vi "Compile Analog Replay Voltage Scaling.vi"(7 "DAC bipolar range":dbl, 8 "error in (no error)":errorcluster, 11 "Item Ref in":T1 format="%.0x") -> (0 "error out":errorcluster, 1 "intercept (b)":fxp<+/-,18,3>, 2 "slope (m)":fxp<+,18,6>, 3 "Item Ref out":T1 format="%.0x")   [LabVIEW 2019, in "Engine Simulation Toolkit System Explorer.lvlib"]
uses:
  Engine Simulation Toolkit System Explorer.lvlib
  <vilib>/NI VeriStand/Custom Device API/Custom Device Item Ref.ctl
  Shared/Properties.vi
  <vilib>/NI VeriStand/Custom Device API/Get Item Property (Double).vi
  <vilib>/NI VeriStand/Custom Device API/Custom Device API.lvlib
  Shared/Engine Simulation Toolkit Shared.lvlib
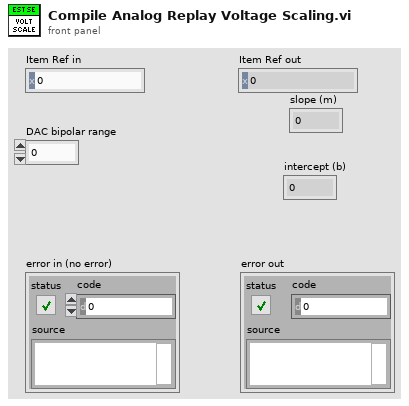
[diagram p1: front panel]
types:
  T1 = typedef "Custom Device API.lvlib/Custom Device Item Ref.ctl" = u64
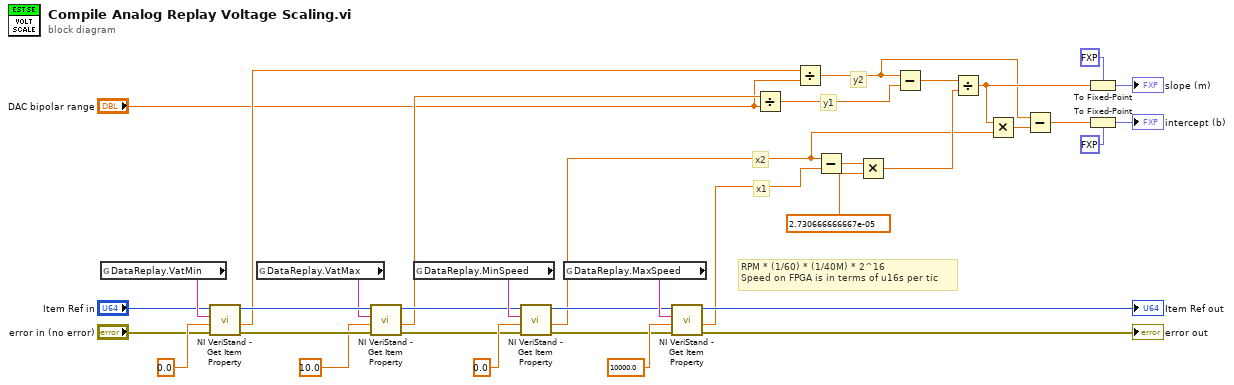
[diagram p0: block diagram]
diagram:
  # "x1"
  # "x2"
  # "y2"
  # "y1"
  # "RPM * (1/60) * (1/40M) * 2^16\nSpeed on FPGA is in terms of u16s per tic"
  n1 = global read "Properties.vi" "DataReplay.VatMin"() -> (w24:string)
  n2 = call-poly <vilib>:"NI VeriStand - Get Item Property.vi"("error in (no error)"="error in (no error)", "Default Value"=0.0, "Property Name"=w24, "Item Ref in"="Item Ref in") -> ("error out"=w23:errorcluster, "Value"=w7:dbl, "Item Ref out"=w22:T1)  [unwired: 4 in, 1 out]
  n3 = global read "Properties.vi" "DataReplay.VatMax"() -> (w20:string)
  n4 = call-poly <vilib>:"NI VeriStand - Get Item Property.vi"("error in (no error)"=w23, "Default Value"=10.0, "Property Name"=w20, "Item Ref in"=w22) -> ("error out"=w12:errorcluster, "Value"=w6:dbl, "Item Ref out"=w13:T1)  [unwired: 4 in, 1 out]
  n5 = global read "Properties.vi" "DataReplay.MinSpeed"() -> (w18:string)
  n6 = call-poly <vilib>:"NI VeriStand - Get Item Property.vi"("error in (no error)"=w12, "Default Value"=0.0, "Property Name"=w18, "Item Ref in"=w13) -> ("error out"=w14:errorcluster, "Value"=w4:dbl, "Item Ref out"=w15:T1)  [unwired: 4 in, 1 out]
  n7 = global read "Properties.vi" "DataReplay.MaxSpeed"() -> (w17:string)
  n8 = call-poly <vilib>:"NI VeriStand - Get Item Property.vi"("error in (no error)"=w14, "Default Value"=10000.0, "Property Name"=w17, "Item Ref in"=w15) -> ("error out"=→"error out":errorcluster, "Value"=w3:dbl, "Item Ref out"=→"Item Ref out":T1)  [unwired: 4 in, 1 out]
  n9 = Divide(x=w6, y="DAC bipolar range") -> (x/y=w34:dbl)
  n10 = Divide(x=w7, y="DAC bipolar range") -> (x/y=w27:dbl)
  n11 = Subtract(x=w4, y=w3) -> (x-y=w32:dbl)
  n12 = Multiply(x=w32, y=2.730666666667e-05) -> (x*y=w31:dbl)
  n13 = Subtract(x=w27, y=w34) -> (x-y=w33:dbl)
  n14 = Divide(x=w33, y=w31) -> (x/y=w29:dbl)
  n15 = Multiply(x=w29, y=w4) -> (x*y=w28:dbl)
  n16 = Subtract(x=w27, y=w28) -> (x-y=w26:dbl)
  n17 = To Fixed-Point(fixed-point type=fxp<+,18,6> 0.0, number=w29) -> (fixed-point=→"slope (m)":fxp<+,18,6>)
  n18 = To Fixed-Point(fixed-point type=fxp<+/-,18,3> 0.0, number=w26) -> (fixed-point=→"intercept (b)":fxp<+/-,18,3>)
